vi "ECG AF SPI Input 2.vi"() -> ()   [LabVIEW 2017]
uses:
  ECG Data.ctl
  IBP Data.ctl
  Trigger Params.ctl
  Channel Enum.ctl
  <vilib>/Platform/TimedLoop/XDataNode/timing_clust.ctl
  <vilib>/Platform/TimedLoop/XDataNode/nitl_modes.ctl
  <vilib>/Platform/TimedLoop/XDataNode/wakeup.ctl
  Gradient Data.ctl
  All Data.ctl
  <vilib>/rvi/Emulation/niFpgaGetClockAttributes.vi
  <vilib>/rvi/Emulation/niFpgaSctlEmulationGetInTimedLoop.vi
  <vilib>/rvi/Emulation/niFpgaEmulationReportErrorSimple.vi
  <vilib>/rvi/DataTransferAndStorage/Container/Common/niFpgaContainerGetUniqueNameForEmu.vi
  <vilib>/rvi/DataTransferAndStorage/Container/Common/niFpgaContainerSetEmuInfo.vi
  <vilib>/rvi/eio/common/nirviEmuReportErrorAndStop.vi
  <vilib>/rvi/Emulation/niFpgaCriticalErrorInLSC.vi
  <vilib>/rvi/Emulation/niFpgaProcessEmulError.vi
  <vilib>/rvi/eio/common/nirviEmuTemplateMethod_errors.vi
  <vilib>/rvi/Analysis/common/codeGenErrors/XNode/niFpgaXNodeCodeGenErrorHandle.vi
  <vilib>/rvi/DataTransferAndStorage/Container/Common/niFpgaContainerExecOnDevCompGetState.vi
  <vilib>/rvi/Emulation/niFpgaEmulationIsFPGAContextNoSignature.vi
  <vilib>/rvi/errors/niFpgaSetErrorForExecOnDevCompSimple.vi
  <vilib>/rvi/FIFO/Fifo_Resource/nirvififoEmulationSetSize.vi
  <vilib>/rvi/FIFO/Fifo_Resource/nirviFifoEmulationQueueMgr.vi
  <instcachedir>/0/nirviFifoEmulationQueueMgr_E5CAEC123FF24DC58D834DCA3CDAA9B5.lvgen/nirviFifoEmulationQueueMgr_E5CAEC123FF24DC58D834DCA3CDAA9B5_002.vi
  <vilib>/rvi/FIFO/Fifo_Resource/nirvififoEmulationDetermineInputValidOut.vi
  <vilib>/rvi/FIFO/Fifo_Resource/nirvififoEmulationCreateLock.vi
  <vilib>/rvi/FIFO/Fifo_Resource/nirvififoEmulationObtainLock.vi
  <vilib>/rvi/FIFO/Fifo_Resource/nirvififoEmulationReleaseLock.vi
  <vilib>/rvi/occurrence/nirviWaitOnOccurrenceBase.vi
  <vilib>/rvi/errors/nirviReportUnexpectedCaseInternalError.vi
  <vilib>/rvi/errors/nirviReportUnexpectedCaseInternalError (U32).vi
  <vilib>/Utility/error.llb/Clear Errors.vi
  <vilib>/rvi/interface/RandomDataEmulation/niFpgaRandomDataHandleErrors.vi
  <instcachedir>/0/nirviFifoEmulationQueueMgr_E5CAEC123FF24DC58D834DCA3CDAA9B5.lvgen/nirviFifoEmulationQueueMgr_E5CAEC123FF24DC58D834DCA3CDAA9B5_003.vi
  <vilib>/Platform/TimedLoop/XDataNode/XDataNode.xnode
  <vilib>/rvi/LocalResourceManager/LocalResourceManager.xnode
  <vilib>/eio/EIONode/EIONode.xnode
  <vilib>/eio/EIOMethodNode/EIOMethodNode.xnode
  <vilib>/rvi/Analysis/measure/butterworth/XNode/niFpgaButterworthFilter.xnode
  <vilib>/rvi/Analysis/measure/LMRsmpl/XNode/niFPGA Rational Resampler.xnode
  <vilib>/rvi/DataTransferAndStorage/Container/XNode/niFpgaContainer.xnode
  <vilib>/rvi/FIFO/Fifo_Resource/niFpgaFifoEmulationRefIn.vi
  <vilib>/Platform/TimedLoop/XDataNode/XDNodeRunTimeDep.lvlib
panel:
  in  "Invert PWM IBP":bool
  in  "Invert PWM ECG":bool
  in  "IBP1":T1={"Scale"=1.0, "Offset"=0.0}
  in  "IBP0":T1={"Scale"=1.0, "Offset"=0.0}
  in  "IBP Filter":bool
  in  "Offset":cluster{"X":i16, "Y":i16, "Z":i16}
  in  "Beta IBP":fxp<+/-,32,-16>
  out "IPB0 In":i16
  out "IBP1 In":i16
  out "IPB0 Out":i16
  out "IBP1 Out":i16
  in  "ECG Scale":i16=1 min=1 max=100 step=1
  out "LL Out":i16
  out "LA Out":i16
  out "RA Out":i16
  out "LL In":i16
  out "LA In":i16
  out "RA In":i16
  in  "HPF":bool
  in  "Trigger":T2
  out "IBP Data":T4
  out "ECG Data":T5
  in  "Stop":bool
  in  "Reset":bool
  out "Send":bool
  out "WeightSum":fxp<+/-,33,19> format="%.20g"
  out "BetaProduct":fxp<+/-,32,-1> format="%.33g"
  out "Loop Time":u32
  in  "Filter Size":i16
  out "I In":i16
  out "II In":i16
  out "III In":i16
  out "aVR In":i16
  out "aVL In":i16
  out "aVF In":i16
  out "V1 In":i16
  out "V2 In":i16
  out "V3 In":i16
  out "V4 In":i16
  out "V5 In":i16
  out "V6 In":i16
  out "V4 Out":i16
  out "V5 Out":i16
  out "Trigger Out":i16
  out "IBP2":i16
  out "IBP1":i16
  out "IBP0":i16
  in  "Start":bool
  in  "Beta ECG":fxp<+/-,32,-16>
  out "V3 Out":i16
  out "V2 Out":i16
  out "V1 Out":i16
  out "aVF Out":i16
  out "aVL Out":i16
  out "aVR Out":i16
  out "III Out":i16
  out "II Out":i16
  out "I Out":i16
  out "V6":i16
  out "V5":i16
  out "V4":i16
  out "V3":i16
  out "V2":i16
  out "V1":i16
  out "LL":i16
  out "LA":i16
  out "Actual Loop Rate (Ticks)":u32
  out "Late? Latched":bool
  out "RA":i16
  in  "Loop Rate (Ticks)":u32=4000
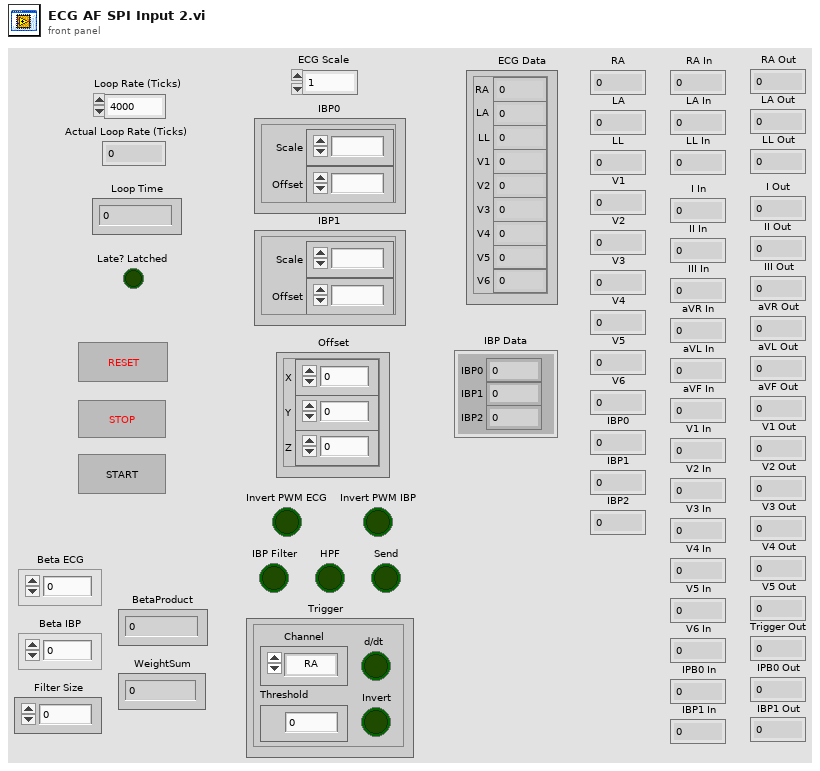
[diagram p1: front panel]
types:
  T1 = cluster{"Scale":fxp<+/-,16,5>, "Offset":fxp<+/-,16,16>}
  T2 = typedef "Trigger Params.ctl" = cluster{"Channel":T3, "Threshold":i16, "d/dt":bool, "Invert":bool}
  T3 = typedef "Channel Enum.ctl" = enum16{"RA", "LA", "LL", "V1", "V2", "V3", "V4", "V5", "V6", "I", "II", "III", "aVR", "aVL", "aVF", "Vw", "IBP1", "IBP2"}
  T4 = typedef "IBP Data.ctl" = cluster{"IBP0":fxp<+/-,16,16>, "IBP1":fxp<+/-,16,16>, "IBP2":fxp<+/-,16,16>}
  T5 = typedef "ECG Data.ctl" = cluster{"RA":fxp<+/-,16,16>, "LA":fxp<+/-,16,16>, "LL":fxp<+/-,16,16>, "V1":fxp<+/-,16,16>, "V2":fxp<+/-,16,16>, "V3":fxp<+/-,16,16>, "V4":fxp<+/-,16,16>, "V5":fxp<+/-,16,16>, "V6":fxp<+/-,16,16>}
  T6 = typedef "XDNodeRunTimeDep.lvlib/timing_clust.ctl" = cluster{"Expected End [f-1]":u64, "Actual End [f-1]":u64, "Finished Late? [f-1]":bool, "Expected End [i-1]":u64, "Actual End [i-1]":u64, "Finished Late? [i-1]":bool, "Expected Start [i]":u64, "Actual Start [i]":u64, "Expected Start [f]":u64, "Actual Start [f]":u64, "Source Name":string, "Structure Name":string, "Period":i64, "Deadline":i64, "Offset":i64, "Start":i64, "Priority":i32, "Timeout":i32, "Mode":T7, "Wakeup Reason":T8, "Error":errorcluster, "Source Type":string, "Secondary Source Type":string, "Global End Time":u64, "Global Start Time":u64, "Frame Duration":u64, "Iteration Duration":u64, "Assigned CPU":i32, "I/O Scan Engine Mode":u32}
  T7 = typedef "XDNodeRunTimeDep.lvlib/nitl_modes.ctl" = enum32{"No Change", "Process missed periods, maintain original phase", "Discard missed periods, maintain original phase", "Process missed periods, ignore original phase", "Discard missed periods, ignore original phase"}
  T8 = typedef "XDNodeRunTimeDep.lvlib/wakeup.ctl" = enum32{"Normal", "Aborted", "Asynchronous wakeup", "Timing source error", "Timed loop error", "Timeout"}
  T9 = typedef "Memory Block Channels.ctl" = cluster{"RA":T10, "LA":T10, "LL":T10, "V1":T10, "V2":T10, "V3":T10, "IBP0":T10, "IBP1":T10}
  T10 = typedef "MemoryBlocks.ctl" = cluster{"Taps":refnum<k21>, "Weights":refnum<k21>, "IO Weights":refnum<k21>, "IO Taps":refnum<k21>}
  T11 = cluster{"ECG":cluster{"RA":fxp<+/-,16,16>, "LA":fxp<+/-,16,16>, "LL":fxp<+/-,16,16>, "V1":fxp<+/-,16,16>, "V2":fxp<+/-,16,16>, "V3":fxp<+/-,16,16>, "V4":fxp<+/-,16,16>, "V5":fxp<+/-,16,16>, "V6":fxp<+/-,16,16>}, "Gradients":cluster{"X":fxp<+/-,16,16>, "Y":fxp<+/-,16,16>, "Z":fxp<+/-,16,16>}, "IBP":cluster{"IBP0":fxp<+/-,16,16>, "IBP1":fxp<+/-,16,16>, "IBP2":fxp<+/-,16,16>}}
  T12 = cluster{"BetaProduct":fxp<+/-,32,-1>, "WeightSum":fxp<+/-,33,19>}
  T13 = typedef "ECG Leads.ctl" = cluster{"RA":i16, "LA":i16, "LL":i16, "V1":i16, "V2":i16, "V3":i16, "V4":i16, "V5":i16, "Trigger":i16, "I":i16, "II":i16, "III":i16, "aVR":i16, "aVL":i16, "aVF":i16, "Vw":i16}
  T14 = cluster{"X":fxp<+/-,16,16>, "Y":fxp<+/-,16,16>, "Z":fxp<+/-,16,16>}
  T15 = cluster{"IBP0":fxp<+/-,16,16>, "IBP1":fxp<+/-,16,16>, "IBP2":fxp<+/-,16,16>}
  T16 = typedef "All Data.ctl" = cluster{"ECG":T5, "Gradients":T17, "IBP":T4}
  T17 = typedef "Gradient Data.ctl" = cluster{"X":fxp<+/-,16,16>, "Y":fxp<+/-,16,16>, "Z":fxp<+/-,16,16>}
  T18 = cluster{"[0]":fxp<+/-,16,16>, "[1]":fxp<+/-,16,16>, "[2]":fxp<+/-,16,16>}
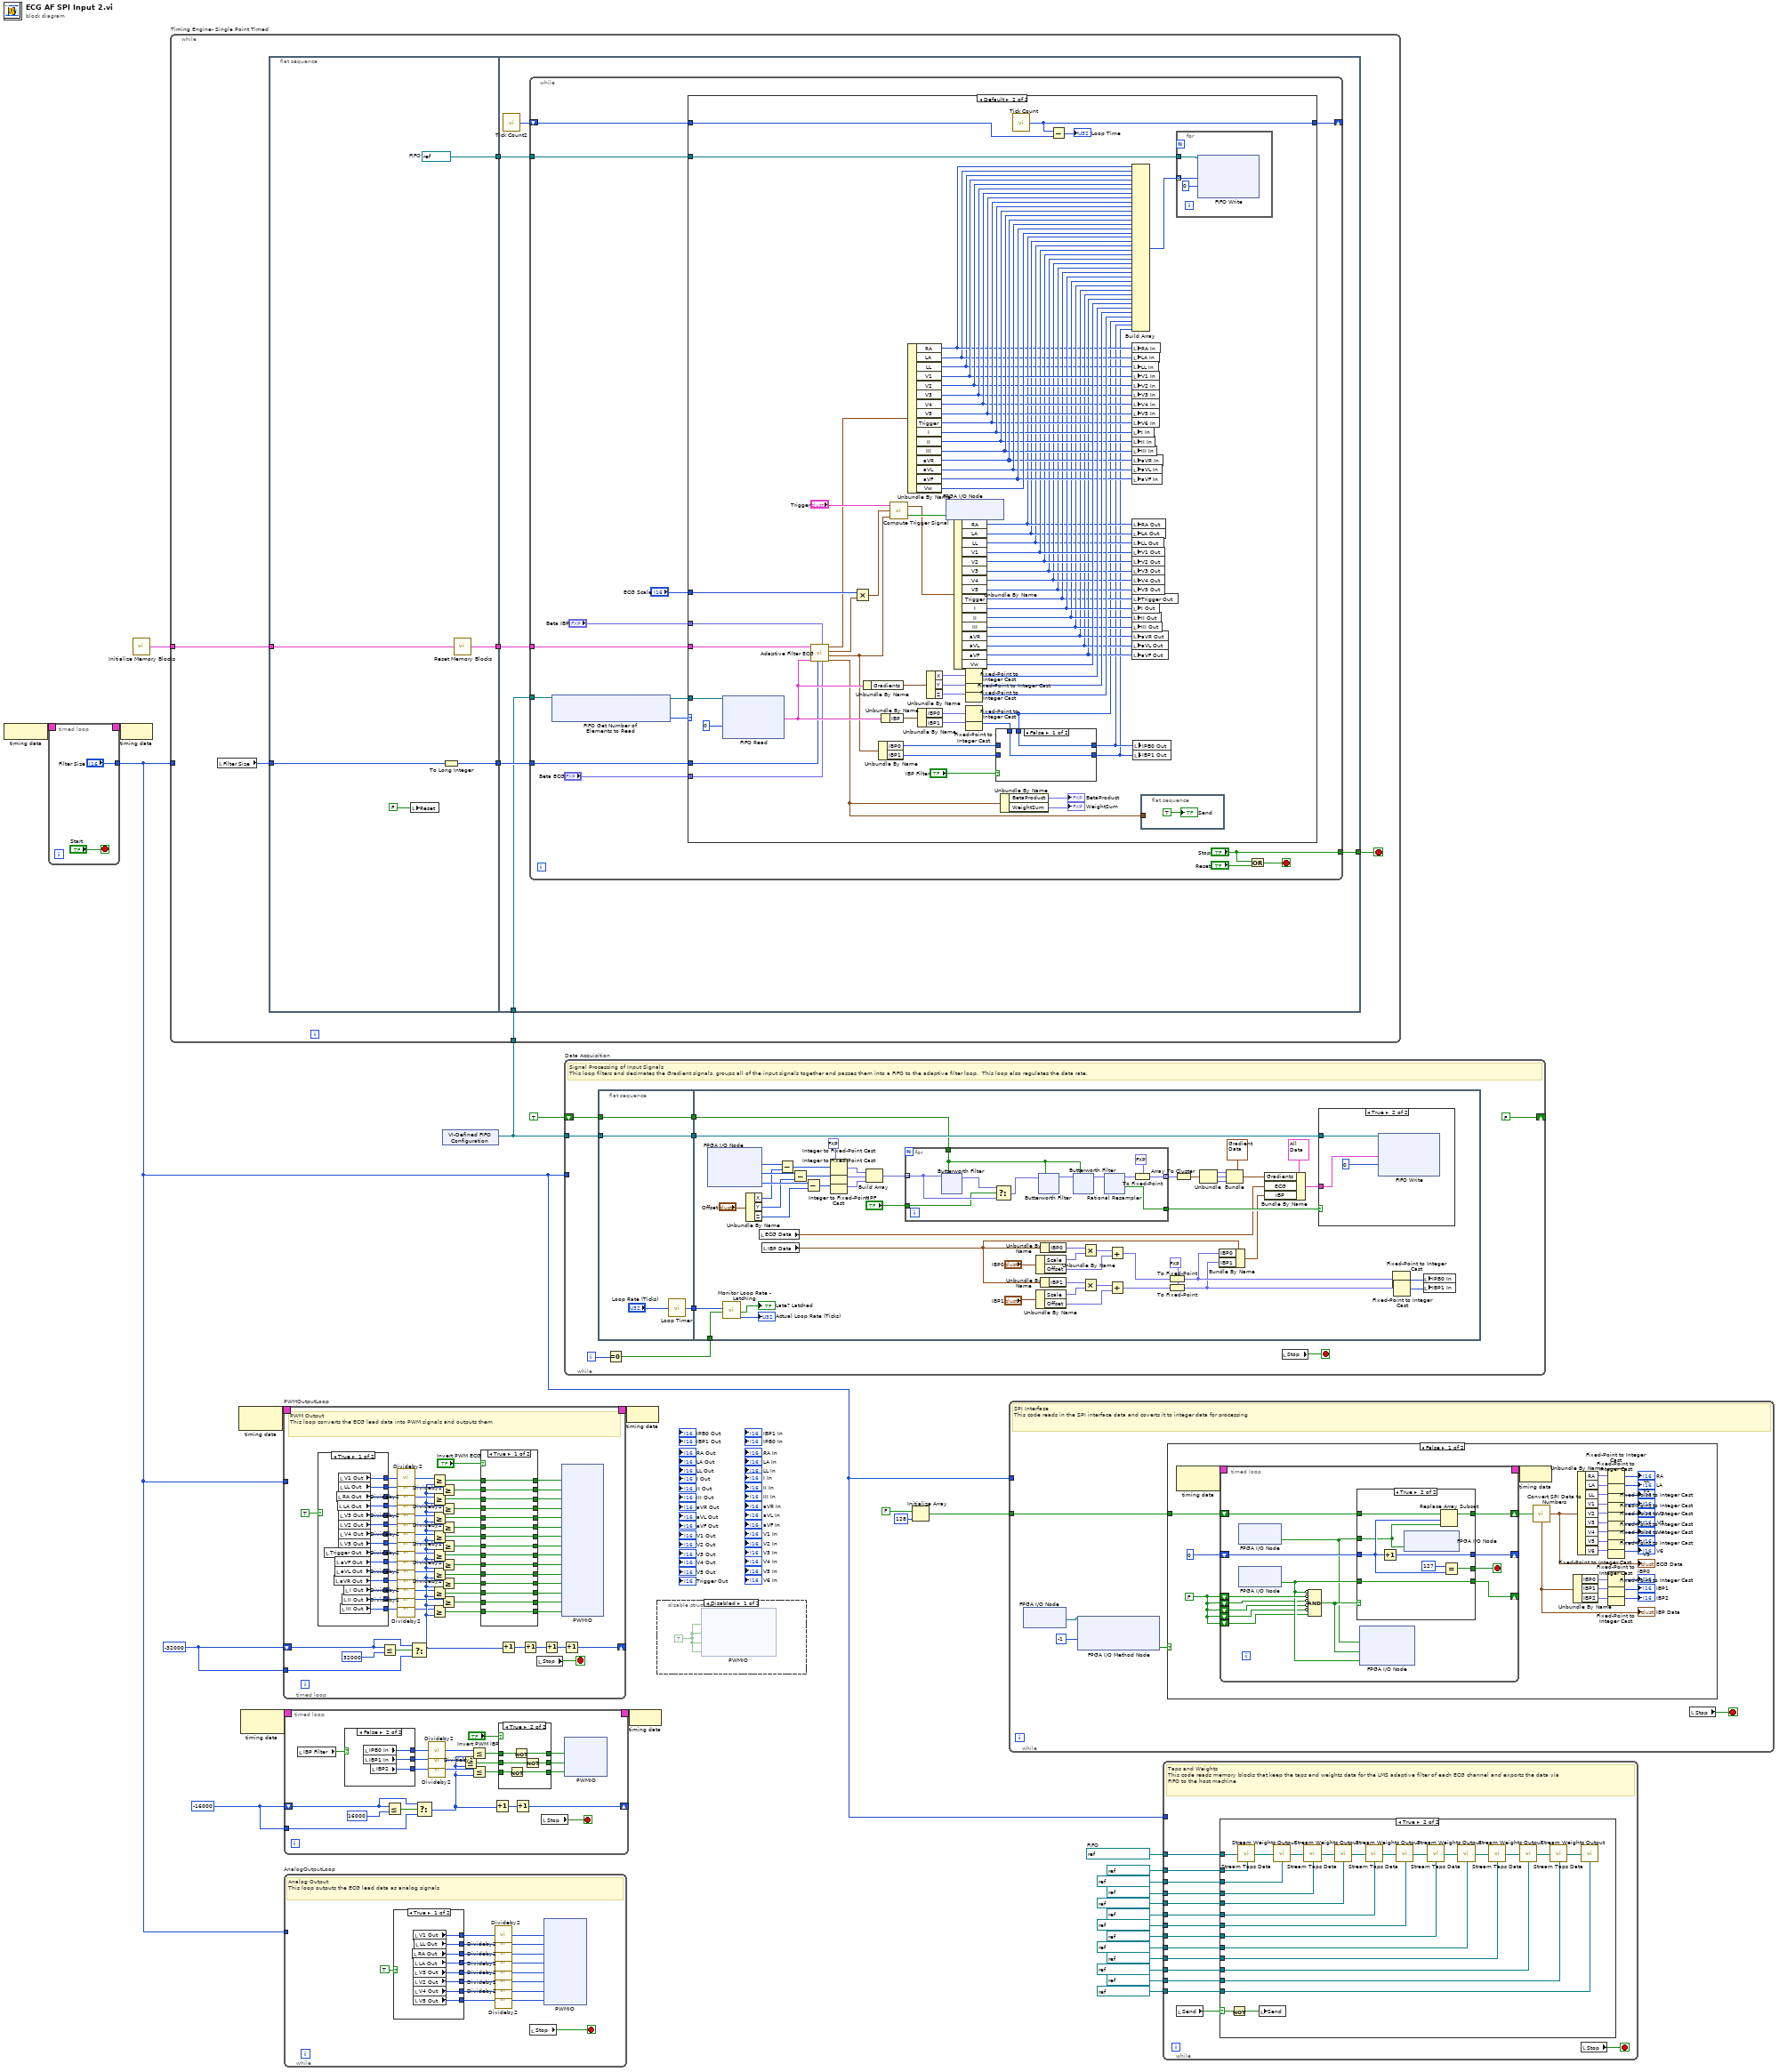
[diagram p0: block diagram]
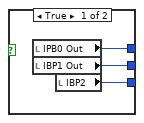
[diagram p4: hidden frame]
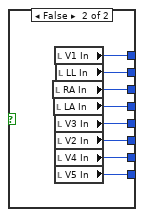
[diagram p7: hidden frame]
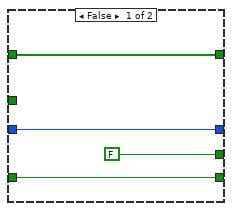
[diagram p8: hidden frame]
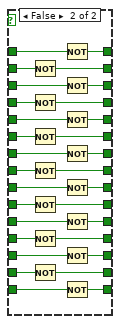
[diagram p10: hidden frame]
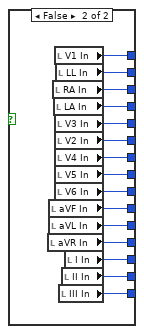
[diagram p11: hidden frame]
diagram:
  w1 = i16 -16000
  w10 = refnum<k21> "FIFO Filter Specs"  # FIFO
  w26 = i16 -32000
  n1 = node-c288 ("Input Node")() -> (w7:T6)
  n2 = timed-loop "initWait" {
    timing: w7 -> [_]
    timing-out: [_] -> w6
    tunnel: ["Filter Size"] -> w5
    stop <- "Start" stop-if-true
  }
  n3 = node-c288 ("Output Node")(w6) -> ()
  n4 = call "Initialize Memory Blocks.vi"() -> ("Memory"=w9:T9)
  n5 = node-c288 ("Input Node")() -> (w28:T6)  [unwired: 1 in]
  n6 = node-c288() -> (w3:T6)  [unwired: 1 in]
  n7 = timed-loop "PWMOutputLoop" {
    timing: w28 -> [_]
    timing-out: [_] -> w27
    shift-right: [w95] -> _
    shift-left: w26 -> [w102]
    tunnel: w26 -> [w100]
    tunnel: w5 -> [_]
    stop <- w72 stop-if-true
    # "PWM Output\nThis loop converts the ECG lead data into PWM signals and outputs them"
    n8 = case shown="True" TRUE {
      tunnel: [w164 w179] -> w98
      tunnel: [w163 w178] -> w97
      tunnel: [w162 w177] -> w91
      tunnel: [w161 w176] -> w92
      tunnel: [w160 w175] -> w88
      tunnel: [w159 w174] -> w87
      tunnel: [w158 w173] -> w89
      tunnel: [w157 w172] -> w90
      tunnel: [w156 w171] -> w86
      tunnel: [w155 w170] -> w78
      tunnel: [w154 w169] -> w77
      tunnel: [w153 w168] -> w76
      tunnel: [w152 w167] -> w71
      tunnel: [w151 w166] -> w70
      tunnel: [w150 w165] -> w69
      frame True {
        n9 = local read "Trigger Out"() -> (w156:i16)
        n10 = local read "aVR Out"() -> (w153:i16)
        n11 = local read "aVF Out"() -> (w155:i16)
        n12 = local read "aVL Out"() -> (w154:i16)
        n13 = local read "RA Out"() -> (w161:i16)
        n14 = local read "LA Out"() -> (w162:i16)
        n15 = local read "V1 Out"() -> (w164:i16)
        n16 = local read "V3 Out"() -> (w157:i16)
        n17 = local read "V2 Out"() -> (w158:i16)
        n18 = local read "V4 Out"() -> (w160:i16)
        n19 = local read "V5 Out"() -> (w159:i16)
        n20 = local read "LL Out"() -> (w163:i16)
        n21 = local read "III Out"() -> (w150:i16)
        n22 = local read "II Out"() -> (w151:i16)
        n23 = local read "I Out"() -> (w152:i16)
      }
      frame False {
        n24 = local read "aVR In"() -> (w168:i16)
        n25 = local read "aVF In"() -> (w170:i16)
        n26 = local read "aVL In"() -> (w169:i16)
        n27 = local read "RA In"() -> (w176:i16)
        n28 = local read "LA In"() -> (w177:i16)
        n29 = local read "V1 In"() -> (w179:i16)
        n30 = local read "V3 In"() -> (w172:i16)
        n31 = local read "V2 In"() -> (w173:i16)
        n32 = local read "V4 In"() -> (w175:i16)
        n33 = local read "V5 In"() -> (w174:i16)
        n34 = local read "V6 In"() -> (w171:i16)
        n35 = local read "LL In"() -> (w178:i16)
        n36 = local read "III In"() -> (w165:i16)
        n37 = local read "II In"() -> (w166:i16)
        n38 = local read "I In"() -> (w167:i16)
      }
    }
    n39 = Less Or Equal?(x=w102, y=i16 32000 ("Period")) -> (x <= y?=w103:bool)
    n40 = call "Divideby2.vi"("Input"=w98) -> ("Output"=w94:i16)
    n41 = call "Divideby2.vi"("Input"=w97) -> ("Output"=w93:i16)
    n42 = call "Divideby2.vi"("Input"=w92) -> ("Output"=w79:i16)
    n43 = call "Divideby2.vi"("Input"=w91) -> ("Output"=w80:i16)
    n44 = call "Divideby2.vi"("Input"=w90) -> ("Output"=w81:i16)
    n45 = call "Divideby2.vi"("Input"=w89) -> ("Output"=w82:i16)
    n46 = call "Divideby2.vi"("Input"=w88) -> ("Output"=w83:i16)
    n47 = call "Divideby2.vi"("Input"=w87) -> ("Output"=w84:i16)
    n48 = call "Divideby2.vi"("Input"=w86) -> ("Output"=w85:i16)
    n49 = call "Divideby2.vi"("Input"=w78) -> ("Output"=w75:i16)
    n50 = call "Divideby2.vi"("Input"=w77) -> ("Output"=w74:i16)
    n51 = call "Divideby2.vi"("Input"=w76) -> ("Output"=w73:i16)
    n52 = call "Divideby2.vi"("Input"=w71) -> ("Output"=w66:i16)
    n53 = call "Divideby2.vi"("Input"=w70) -> ("Output"=w67:i16)
    n54 = call "Divideby2.vi"("Input"=w69) -> ("Output"=w65:i16)
    n55 = Select(t=w102, s=w103, f=w100) -> (s? t:f=w68:i16)
    n56 = Greater Or Equal?(x=w94, y=w68) -> (x >= y?=w62:bool)
    n57 = Greater Or Equal?(x=w79, y=w68) -> (x >= y?=w60:bool)
    n58 = Greater Or Equal?(x=w81, y=w68) -> (x >= y?=w58:bool)
    n59 = Greater Or Equal?(x=w83, y=w68) -> (x >= y?=w56:bool)
    n60 = Greater Or Equal?(x=w85, y=w68) -> (x >= y?=w54:bool)
    n61 = Greater Or Equal?(x=w74, y=w68) -> (x >= y?=w52:bool)
    n62 = Greater Or Equal?(x=w66, y=w68) -> (x >= y?=w50:bool)
    n63 = Greater Or Equal?(x=w65, y=w68) -> (x >= y?=w48:bool)
    n64 = Greater Or Equal?(x=w93, y=w68) -> (x >= y?=w61:bool)
    n65 = Greater Or Equal?(x=w80, y=w68) -> (x >= y?=w59:bool)
    n66 = Greater Or Equal?(x=w82, y=w68) -> (x >= y?=w57:bool)
    n67 = Greater Or Equal?(x=w84, y=w68) -> (x >= y?=w55:bool)
    n68 = Greater Or Equal?(x=w75, y=w68) -> (x >= y?=w53:bool)
    n69 = Greater Or Equal?(x=w73, y=w68) -> (x >= y?=w51:bool)
    n70 = Greater Or Equal?(x=w67, y=w68) -> (x >= y?=w49:bool)
    n71 = case shown="True" "Invert PWM ECG" {
      tunnel: w62 -> [w119 w149]
      tunnel: w61 -> [w118 w148]
      tunnel: w60 -> [w117 w147]
      tunnel: w59 -> [w116 w146]
      tunnel: w58 -> [w115 w145]
      tunnel: w57 -> [w114 w144]
      tunnel: w56 -> [w113 w143]
      tunnel: w55 -> [w112 w142]
      tunnel: w54 -> [w111 w141]
      tunnel: w53 -> [w110 w140]
      tunnel: w52 -> [w109 w139]
      tunnel: w51 -> [w108 w138]
      tunnel: w50 -> [w107 w137]
      tunnel: w49 -> [w106 w136]
      tunnel: w48 -> [w105 w135]
      tunnel: [w119 w134] -> w47
      tunnel: [w118 w133] -> w46
      tunnel: [w117 w132] -> w45
      tunnel: [w116 w131] -> w44
      tunnel: [w115 w130] -> w43
      tunnel: [w114 w129] -> w42
      tunnel: [w113 w128] -> w41
      tunnel: [w112 w127] -> w40
      tunnel: [w111 w126] -> w39
      tunnel: [w110 w125] -> w38
      tunnel: [w109 w124] -> w37
      tunnel: [w108 w123] -> w36
      tunnel: [w107 w122] -> w35
      tunnel: [w106 w121] -> w34
      tunnel: [w105 w120] -> w33
      frame True {
      }
      frame False {
        n72 = Not(x=w148) -> (.not. x?=w133:bool)
        n73 = Not(x=w146) -> (.not. x?=w131:bool)
        n74 = Not(x=w144) -> (.not. x?=w129:bool)
        n75 = Not(x=w142) -> (.not. x?=w127:bool)
        n76 = Not(x=w140) -> (.not. x?=w125:bool)
        n77 = Not(x=w138) -> (.not. x?=w123:bool)
        n78 = Not(x=w136) -> (.not. x?=w121:bool)
        n79 = Not(x=w149) -> (.not. x?=w134:bool)
        n80 = Not(x=w147) -> (.not. x?=w132:bool)
        n81 = Not(x=w145) -> (.not. x?=w130:bool)
        n82 = Not(x=w143) -> (.not. x?=w128:bool)
        n83 = Not(x=w141) -> (.not. x?=w126:bool)
        n84 = Not(x=w139) -> (.not. x?=w124:bool)
        n85 = Not(x=w137) -> (.not. x?=w122:bool)
        n86 = Not(x=w135) -> (.not. x?=w120:bool)
      }
    }
    n87 = Increment(x=w68) -> (x+1=w101:i16)
    n88 = Increment(x=w101) -> (x+1=w99:i16)
    n89 = local read "Stop"() -> (w72:bool)
    n90 = Increment(x=w99) -> (x+1=w96:i16)
    n91 = xnode ("PWMIO")("V1"=w47, "LL"=w46, "RA"=w45, "LA"=w44, "V3"=w43, "V2"=w42, "V4"=w41, "V5"=w40, "V6"=w39, "aVF"=w38, "aVL"=w37, "aVR"=w36, "I"=w35, "II"=w34, "III"=w33) -> ()  [unwired: 15 in, 15 out]
    n92 = Increment(x=w96) -> (x+1=w95:i16)
  }
  n93 = while "AnalogOutputLoop" {
    tunnel: w5 -> [_]
    stop <- w196 stop-if-true
    # "Analog Output\nThis loop outputs the ECG lead data as analog signals"
    n94 = case shown="True" TRUE {
      tunnel: [w207 w215] -> w198
      tunnel: [w206 w214] -> w197
      tunnel: [w205 w213] -> w199
      tunnel: [w200 w212] -> w187
      tunnel: [w201 w211] -> w186
      tunnel: [w202 w210] -> w185
      tunnel: [w203 w209] -> w184
      tunnel: [w204 w208] -> w183
      frame True {
        n95 = local read "RA Out"() -> (w202:i16)
        n96 = local read "LA Out"() -> (w201:i16)
        n97 = local read "V1 Out"() -> (w204:i16)
        n98 = local read "V3 Out"() -> (w200:i16)
        n99 = local read "V2 Out"() -> (w205:i16)
        n100 = local read "V4 Out"() -> (w207:i16)
        n101 = local read "V5 Out"() -> (w206:i16)
        n102 = local read "LL Out"() -> (w203:i16)
      }
      frame False {
        n103 = local read "RA In"() -> (w210:i16)
        n104 = local read "LA In"() -> (w211:i16)
        n105 = local read "V1 In"() -> (w208:i16)
        n106 = local read "V3 In"() -> (w212:i16)
        n107 = local read "V2 In"() -> (w213:i16)
        n108 = local read "V4 In"() -> (w215:i16)
        n109 = local read "V5 In"() -> (w214:i16)
        n110 = local read "LL In"() -> (w209:i16)
      }
    }
    n111 = call "Divideby2.vi"("Input"=w183) -> ("Output"=w195:i16)
    n112 = call "Divideby2.vi"("Input"=w184) -> ("Output"=w194:i16)
    n113 = call "Divideby2.vi"("Input"=w185) -> ("Output"=w193:i16)
    n114 = call "Divideby2.vi"("Input"=w186) -> ("Output"=w192:i16)
    n115 = call "Divideby2.vi"("Input"=w187) -> ("Output"=w191:i16)
    n116 = call "Divideby2.vi"("Input"=w199) -> ("Output"=w190:i16)
    n117 = call "Divideby2.vi"("Input"=w198) -> ("Output"=w189:i16)
    n118 = call "Divideby2.vi"("Input"=w197) -> ("Output"=w188:i16)
    n119 = local read "Stop"() -> (w196:bool)
    n120 = xnode ("PWMIO")("ECG0"=w195, "ECG1"=w194, "ECG2"=w193, "ECG3"=w192, "ECG4"=w191, "ECG5"=w190, "ECG6"=w189, "ECG7"=w188) -> ()  [unwired: 8 in, 8 out]
  }
  n121 = timed-loop {
    timing: w3 -> [_]
    timing-out: [_] -> w2
    shift-right: [w223] -> _
    shift-left: w1 -> [w229]
    tunnel: w1 -> [w227]
    stop <- w228 stop-if-true
    n122 = local read "IBP Filter"() -> (w226:bool)
    n123 = case shown="False" w226 {
      tunnel: [w249 w252] -> w234
      tunnel: [w248 w251] -> w233
      tunnel: [w247 w250] -> w232
      frame True {
        n124 = local read "IPB0 Out"() -> (w249:i16)
        n125 = local read "IBP1 Out"() -> (w248:i16)
        n126 = local read "IBP2"() -> (w247:i16)
      }
      frame False {
        n127 = local read "IPB0 In"() -> (w252:i16)
        n128 = local read "IBP1 In"() -> (w251:i16)
        n129 = local read "IBP2"() -> (w250:i16)
      }
    }
    n130 = Less Or Equal?(x=w229, y=i16 16000 ("Period")) -> (x <= y?=w231:bool)
    n131 = Select(t=w229, s=w231, f=w227) -> (s? t:f=w225:i16)
    n132 = call "Divideby2.vi"("Input"=w234) -> ("Output"=w237:i16)
    n133 = call "Divideby2.vi"("Input"=w233) -> ("Output"=w236:i16)
    n134 = call "Divideby2.vi"("Input"=w232) -> ("Output"=w235:i16)
    n135 = Less Or Equal?(x=w236, y=w225) -> (x <= y?=w220:bool)
    n136 = Less Or Equal?(x=w237, y=w225) -> (x <= y?=w221:bool)
    n137 = Less Or Equal?(x=w235, y=w225) -> (x <= y?=w219:bool)
    n138 = Increment(x=w225) -> (x+1=w224:i16)
    n139 = case shown="True" "Invert PWM IBP" {
      tunnel: w221 -> [w240 w246]
      tunnel: w220 -> [w239 w245]
      tunnel: w219 -> [w238 w244]
      tunnel: [w240 w243] -> w218
      tunnel: [w239 w242] -> w217
      tunnel: [w238 w241] -> w216
      frame False {
      }
      frame True {
        n140 = Not(x=w244) -> (.not. x?=w241:bool)
        n141 = Not(x=w246) -> (.not. x?=w243:bool)
        n142 = Not(x=w245) -> (.not. x?=w242:bool)
      }
    }
    n143 = Increment(x=w224) -> (x+1=w223:i16)
    n144 = local read "Stop"() -> (w228:bool)
    n145 = xnode ("PWMIO")("IBP0"=w218, "IBP1"=w217, "IBP2"=w216) -> ()  [unwired: 3 in, 3 out]
  }
  n146 = xnode "VI-Defined FIFO Configuration"() -> ("FIFO Out"=w8:refnum<k21>)
  n147 = while "Timing Engine- Single Point Timed" {
    tunnel: w9 -> [w257]
    tunnel: w8 -> [w256]
    tunnel: w5 -> [_]
    stop <- w258 stop-if-true
    n148 = local read "Filter Size"() -> (w255:i16)
    n149 = flat-sequence "MainSeq" {
      tunnel: [w267] -> w261
      tunnel: [w266] -> w260
      tunnel: [w265] -> w259
      tunnel: w257 -> [w264]
      tunnel: w255 -> [w263]
      tunnel: w261 -> [w273]
      tunnel: w260 -> [w272]
      tunnel: w259 -> [w271]
      tunnel: [w269] -> w258
      tunnel: w256 -> [w268]
      frame #0 {
        w267 = refnum<k21> "FIFO"  # FIFO
        n150 = local write "Reset"(FALSE ("Reset")) -> ()
        n151 = To Long Integer(number=w263) -> (32bit integer=w266:i32)
        n152 = call "Reset Memory Blocks.vi"("Memory Blocks In"=w264) -> ("Memory Blocks Out"=w265:T9)  [unwired: 1 in]
      }
      frame #1 {
        n153 = call "Tick Count2"() -> ("Tick Count(uSec)"=w270:u32)
        n154 = while {
          tunnel: w268 -> [w287]
          tunnel: w273 -> [w283]
          tunnel: w272 -> [w282]
          tunnel: w271 -> [w276]
          shift-right: [w281] -> _
          shift-left: w270 -> [w280]
          tunnel: ["Stop"] -> w269
          stop <- w278 stop-if-true
          n155 = xnode ("FIFO Get Number of Elements to Read")("FIFO In"=w287) -> ("Number of Elements to Read"=w286:u32, "FIFO Out"=w285:refnum<k21>)
          n156 = case shown="Default" w286 {
            tunnel: w285 -> [_ w360]
            tunnel: "Beta ECG" -> [_ w312]
            tunnel: w283 -> [_ w358]
            tunnel: w282 -> [_ w313]
            tunnel: w280 -> [w288 w322]
            tunnel: [w288 w323] -> w281
            tunnel: w276 -> [_ w319]
            tunnel: "ECG Scale" -> [_ w302]
            tunnel: "Beta IBP" -> [_ w299]
            frame 0 {
            }
            frame Default {
              n157 = xnode ("FIFO Read")("Timeout"=0, "FIFO In"=w360) -> ("Element"=w315:T11)  [unwired: 2 out]
              n158 = call "Adaptive Filter ECG.vi"("Beta"=w312, "Beta IBP"=w299, "Filter Length"=w313, "Data in"=w315, "Memory Blocks In"=w319) -> ("Data"=w314:T12, "IBP Out"=w298:cluster{"IBP0":i16, "IBP1":i16}, "Filtered Leads"=w303:T13, "Raw Leads"=w300:T13)  [unwired: 3 in]
              n159 = Multiply(x=w302, y=w303) -> (x*y=w301:T13)
              n160 = Unbundle By Name(w315) -> ("Gradients"=w318:T14)
              n161 = Unbundle By Name(w298) -> ("IBP0"=w294:i16, "IBP1"=w295:i16)
              n162 = Unbundle By Name(w315) -> ("IBP"=w317:T15)
              n163 = call "Compute Trigger Signal.vi"("IBP Out"=w298, "Filtered Leads"=w301, "Trigger"="Trigger") -> ("Trigger Out"=w310:bool, "Leads Out"=w289:T13)
              n164 = Unbundle By Name(w300) -> ("RA"=w306:i16, "LA"=w305:i16, "LL"=w304:i16, "V1"=w337:i16, "V2"=w338:i16, "V3"=w339:i16, "V4"=w340:i16, "V5"=w341:i16, "Trigger"=w342:i16, "I"=w343:i16, "II"=w344:i16, "III"=w345:i16, "aVR"=w346:i16, "aVL"=w347:i16, "aVF"=w348:i16, "Vw"=w353:i16)
              n165 = Unbundle By Name(w317) -> ("IBP0"=w316:fxp<+/-,16,16>, "IBP1"=w297:fxp<+/-,16,16>)
              n166 = Unbundle By Name(w318) -> ("X"=w356:fxp<+/-,16,16>, "Y"=w355:fxp<+/-,16,16>, "Z"=w354:fxp<+/-,16,16>)
              n167 = xnode "FPGA I/O Node"("Trigger Out"=w310) -> ()  [unwired: 1 in, 1 out]
              n168 = Unbundle By Name(w289) -> ("RA"=w309:i16, "LA"=w308:i16, "LL"=w307:i16, "V1"=w336:i16, "V2"=w335:i16, "V3"=w334:i16, "V4"=w333:i16, "V5"=w325:i16, "Trigger"=w326:i16, "I"=w332:i16, "II"=w331:i16, "III"=w330:i16, "aVR"=w329:i16, "aVL"=w328:i16, "aVF"=w327:i16, "Vw"=w352:i16)
              n169 = Fixed-Point to Integer Cast(1:w356) -> (0:w351:i16)
              n170 = Fixed-Point to Integer Cast(1:w355) -> (0:w350:i16)
              n171 = Fixed-Point to Integer Cast(1:w354) -> (0:w349:i16)
              n172 = Fixed-Point to Integer Cast(1:w316) -> (0:w290:i16)
              n173 = Fixed-Point to Integer Cast(1:w297) -> (0:w291:i16)
              n174 = case shown="False" "IBP Filter" {
                tunnel: w295 -> [_ w363]
                tunnel: w294 -> [_ w364]
                tunnel: [w361 w364] -> w293
                tunnel: [w362 w363] -> w292
                tunnel: w291 -> [w362 _]
                tunnel: w290 -> [w361 _]
                frame False {
                }
                frame True {
                }
              }
              n175 = Unbundle By Name(w314) -> ("BetaProduct"=→"BetaProduct":fxp<+/-,32,-1>, "WeightSum"=→"WeightSum":fxp<+/-,33,19>)
              n176 = call "Tick Count"() -> ("Tick Count(uSec)"=w323:u32)
              n177 = Subtract(x=w323, y=w322) -> (x-y=→"Loop Time":u32)
              n178 = Build Array(w306, w305, w304, w337, w338, w339, w340, w341, w342, w343, w344, w345, w346, w347, w348, w353, w309, w308, w307, w336, w335, w334, w333, w325, w326, w332, w331, w330, w329, w328, w327, w352, w351, w350, w349, w290, w293, w292) -> (w357:i16[])
              n179 = local write "RA In"(w306) -> ()
              n180 = local write "LA In"(w305) -> ()
              n181 = local write "LL In"(w304) -> ()
              n182 = local write "V1 In"(w337) -> ()
              n183 = local write "V2 In"(w338) -> ()
              n184 = local write "V3 In"(w339) -> ()
              n185 = local write "V4 In"(w340) -> ()
              n186 = local write "V5 In"(w341) -> ()
              n187 = local write "V6 In"(w342) -> ()
              n188 = local write "I In"(w343) -> ()
              n189 = local write "II In"(w344) -> ()
              n190 = local write "III In"(w345) -> ()
              n191 = local write "aVR In"(w346) -> ()
              n192 = local write "aVL In"(w347) -> ()
              n193 = local write "aVF In"(w348) -> ()
              n194 = local write "RA Out"(w309) -> ()
              n195 = local write "LA Out"(w308) -> ()
              n196 = local write "LL Out"(w307) -> ()
              n197 = local write "V1 Out"(w336) -> ()
              n198 = local write "V2 Out"(w335) -> ()
              n199 = local write "V3 Out"(w334) -> ()
              n200 = local write "V4 Out"(w333) -> ()
              n201 = local write "V5 Out"(w325) -> ()
              n202 = local write "Trigger Out"(w326) -> ()
              n203 = local write "I Out"(w332) -> ()
              n204 = local write "II Out"(w331) -> ()
              n205 = local write "III Out"(w330) -> ()
              n206 = local write "aVR Out"(w329) -> ()
              n207 = local write "aVL Out"(w328) -> ()
              n208 = local write "aVF Out"(w327) -> ()
              n209 = local write "IPB0 Out"(w293) -> ()
              n210 = local write "IBP1 Out"(w292) -> ()
              n211 = flat-sequence {
                tunnel: w314 -> [_]
                frame #0 {
                  "Send" <- TRUE ("Send")
                }
              }
              n212 = for {
                tunnel: w358 -> [w368]
                tunnel: w357 -> [w366] mode=indexing
                n213 = xnode ("FIFO Write")("Element"=w366, "Timeout"=0, "FIFO In"=w368) -> ()  [unwired: 2 out]
              }
            }
          }
          n214 = Or(x="Stop", y="Reset") -> (x .or. y?=w278:bool)
        }
      }
    }
  }
  n215 = while "Data Acquisition" {
    tunnel: w8 -> [w376]
    tunnel: w5 -> [_]
    shift-right: [FALSE] -> _
    shift-left: TRUE -> [w371]
    i -> [w374]
    stop <- w372 stop-if-true
    # "Signal Processing of Input Signals\nThis loop filters and decimates the Gradient signals, groups all of the input signals together and passes them into a FIFO to the adaptive filter loop.  This loop also regulates the data rate."
    n216 = flat-sequence "Data Acquisition Sequence" {
      tunnel: ["Loop Rate (Ticks)"] -> w377
      tunnel: w376 -> [w380]
      tunnel: [w380] -> w375
      tunnel: w371 -> [w378]
      tunnel: [w378] -> w370
      tunnel: w377 -> [w430]
      tunnel: w373 -> [w431]
      tunnel: w375 -> [w429]
      tunnel: w370 -> [w408]
      frame #0 {
        n217 = call "Loop Timer"("Count(Ticks)"="Loop Rate (Ticks)") -> ()  [unwired: 1 out]
      }
      frame #1 {
        w393 = fxp<+/-,16,16> 0.0 ("IBP Scale")
        w419 = fxp<+/-,16,16> 0.0 ("fixed-point type")
        n218 = xnode "FPGA I/O Node"() -> ("X Gradient"=w422:i16, "Y Gradient"=w421:i16, "Z Gradient"=w420:i16)  [unwired: 3 in, 3 out]
        n219 = call "Monitor Loop Rate - Latching.vi"("Reset"=w431, "Count(Ticks)"=w430) -> ("Actual Loop Rate (Ticks)"=→"Actual Loop Rate (Ticks)":u32, "Late? (Latched)"=→"Late? Latched":bool)  [unwired: 7 in, 1 out]
        n220 = Unbundle By Name("Offset") -> ("X"=w402:i16, "Y"=w400:i16, "Z"=w398:i16)
        n221 = local read "ECG Data"() -> (w409:T5)
        n222 = local read "IBP Data"() -> (w383:T4)
        n223 = Subtract(x=w422, y=w402) -> (x-y=w403:i16)
        n224 = Subtract(x=w421, y=w400) -> (x-y=w401:i16)
        n225 = Subtract(x=w420, y=w398) -> (x-y=w399:i16)
        n226 = Integer to Fixed-Point Cast(fixed-point type=w419, integer=w403) -> (fixed-point=w424:fxp<+/-,16,16>)
        n227 = Integer to Fixed-Point Cast(fixed-point type=w419, integer=w401) -> (fixed-point=w425:fxp<+/-,16,16>)
        n228 = Integer to Fixed-Point Cast(fixed-point type=w419, integer=w399) -> (fixed-point=w423:fxp<+/-,16,16>)
        n229 = Build Array(w424, w425, w423) -> (w426:fxp<+/-,16,16>[])
        n230 = for {
          tunnel: w426 -> [w435] mode=indexing
          tunnel: [w439] -> w418 mode=indexing
          tunnel: [w440] -> w428
          tunnel: w408 -> [w437]
          tunnel: "HPF" -> [w433]
          n231 = xnode "Butterworth Filter"("input data"=w435, "reset"=w437) -> ("output data"=w436:fxp<+/-,16,16>)  [unwired: 1 in, 1 out]
          n232 = Select(t=w436, s=w433, f=w435) -> (s? t:f=w434:fxp<+/-,16,16>)
          n233 = xnode "Butterworth Filter"("input data"=w434, "reset"=w437) -> ("output data"=w443:fxp<+/-,16,16>)  [unwired: 1 in, 1 out]
          n234 = xnode "Butterworth Filter"("input data"=w443, "reset"=w437) -> ("output data"=w442:fxp<+/-,16,16>)  [unwired: 1 in, 1 out]
          n235 = xnode "Rational Resampler"("input data"=w442) -> ("output data"=w441:fxp<+/-,18,16>, "output valid"=w440:bool)  [unwired: 1 out]
          n236 = To Fixed-Point(fixed-point type=fxp<+/-,16,16> 0.0, number=w441) -> (fixed-point=w439:fxp<+/-,16,16>)
        }
        n237 = Unbundle By Name("IBP0") -> ("Scale"=w391:fxp<+/-,16,5>, "Offset"=w389:fxp<+/-,16,16>)
        n238 = Unbundle By Name("IBP1") -> ("Scale"=w385:fxp<+/-,16,5>, "Offset"=w387:fxp<+/-,16,16>)
        n239 = Unbundle By Name(w383) -> ("IBP0"=w390:fxp<+/-,16,16>)
        n240 = Unbundle By Name(w383) -> ("IBP1"=w386:fxp<+/-,16,16>)
        n241 = Multiply(x=w390, y=w391) -> (x*y=w397:fxp<+/-,32,21>)
        n242 = Multiply(x=w386, y=w385) -> (x*y=w384:fxp<+/-,32,21>)
        n243 = Add(x=w397, y=w389) -> (x+y=w388:fxp<+/-,32,21>)
        n244 = Add(x=w384, y=w387) -> (x+y=w381:fxp<+/-,32,21>)
        n245 = To Fixed-Point(fixed-point type=w393, number=w388) -> (fixed-point=w396:fxp<+/-,16,16>)
        n246 = To Fixed-Point(fixed-point type=w393, number=w381) -> (fixed-point=w394:fxp<+/-,16,16>)
        n247 = Array To Cluster(array=w418) -> (cluster=w417:T18)
        n248 = Unbundle(w417) -> ("[0]"=w415:fxp<+/-,16,16>, "[1]"=w414:fxp<+/-,16,16>, "[2]"=w413:fxp<+/-,16,16>)
        n249 = Bundle By Name(cluster=w383, "IBP0"=w396, "IBP1"=w394) -> (w395:T4)
        n250 = Bundle(cluster=T17 {"X"=0.0, "Y"=0.0, "Z"=0.0} ("Gradients"), "X"=w415, "Y"=w414, "Z"=w413) -> (w411:T17)
        n251 = Bundle By Name(cluster=T16 {"ECG"={"RA"=0.0, "LA"=0.0, "LL"=0.0, "V1"=0.0, "V2"=0.0, "V3"=0.0, "V4"=0.0, "V5"=0.0, "V6"=0.0}, "Gradients"={"X"=0.0, "Y"=0.0, "Z"=0.0}, "IBP"={"IBP0"=0.0, "IBP1"=0.0, "IBP2"=0.0}} ("Data"), "Gradients"=w411, "ECG"=w409, "IBP"=w395) -> (w410:T16)
        n252 = case shown="True" w428 {
          tunnel: w429 -> [_ w523]
          tunnel: w410 -> [_ w521]
          frame False {
          }
          frame True {
            n253 = xnode ("FIFO Write")("Element"=w521, "Timeout"=0, "FIFO In"=w523) -> ()  [unwired: 2 out]
          }
        }
        n254 = Fixed-Point to Integer Cast(1:w396) -> (0:w405:i16)
        n255 = Fixed-Point to Integer Cast(1:w394) -> (0:w406:i16)
        n256 = local write "IPB0 In"(w405) -> ()
        n257 = local write "IBP1 In"(w406) -> ()
      }
    }
    n258 = Equal To 0?(x=w374) -> (x = 0?=w373:bool)
    n259 = local read "Stop"() -> (w372:bool)
  }
  n260 = node-c288 ("Output Node")(w27) -> ()
  n261 = node-c288(w2) -> ()
  n262 = disable-structure shown="Disabled" {
    frame Disabled {
      w524 = TRUE
      n263 = xnode ("PWMIO")("Connector2/DIO2"=w524, "Connector2/DIO3"=w524, "Connector2/DIO4"=w524, "Connector2/DIO5"=w524) -> ()  [unwired: 4 in, 4 out]
    }
    frame Enabled {
    }
  }
  n264 = Initialize Array(FALSE, 128 ("dimension size")) -> (w25:bool[])
  n265 = while {
    tunnel: w25 -> [w526]
    tunnel: w5 -> [_]
    stop <- w525 stop-if-true
    # "SPI Interface\nThis code reads in the SPI interface data and coverts it to integer data for processing"
    n266 = xnode "FPGA I/O Node"() -> ("FPGA I/O Out"=w527:refnum<k21>)  [unwired: 1 in, 1 out]
    n267 = xnode "FPGA I/O Method Node"("FPGA I/O In"=w527, "Timeout"=-1) -> ("Timed Out"=w528:bool)  [unwired: 1 out]
    n268 = case shown="False" w528 {
      tunnel: w526 -> [w561 _]
      frame False {
        w557 = FALSE
        n269 = node-c288() -> (w560:T6)  [unwired: 1 in]
        n270 = timed-loop {
          shift-right: [w573] -> w556
          shift-left: w561 -> [w574]
          timing: w560 -> [_]
          timing-out: [_] -> w559
          shift-right: [w569] -> _
          shift-left: w557 -> [w572]
          shift-right: [w570] -> _
          shift-left: u8 0 -> [w571]
          shift-left: w557 -> [w565]
          shift-left: w557 -> [w564]
          shift-left: w557 -> [w563]
          shift-left: w557 -> [w562]
          stop <- w575 stop-if-true
          n271 = xnode "FPGA I/O Node"() -> ("MOSI"=w566:bool)  [unwired: 1 in, 1 out]
          n272 = xnode "FPGA I/O Node"() -> ("SCLK"=w568:bool)  [unwired: 1 in, 1 out]
          n273 = Compound Arithmetic op=AND(invert w568, invert w572, invert w565, invert w564, invert w563, w562) -> (w567:bool)
          n274 = case shown="True" w567 {
            tunnel: [FALSE w586] -> w575
            tunnel: w574 -> [w576 w585]
            tunnel: [w576 w584] -> w573
            tunnel: w571 -> [w579 w583]
            tunnel: [w579 w582] -> w570
            tunnel: w568 -> [w578 w581]
            tunnel: [w578 w581] -> w569
            tunnel: w566 -> [_ w580]
            frame False {
            }
            frame True {
              n275 = Increment(x=w583) -> (x+1=w582:u8)
              n276 = xnode "FPGA I/O Node"("MOSI Data"=w580) -> ()  [unwired: 1 in, 1 out]
              n277 = Replace Array Subset(array=w585, new element=w580, index=w583) -> (w584:bool[])
              n278 = Equal?(x=u8 127, y=w583) -> (x = y?=w586:bool)
            }
          }
          n279 = xnode "FPGA I/O Node"("MOSI Out"=w566, "SCLK Edge"=w567, "SCLK Out"=w568) -> ()  [unwired: 3 in, 3 out]
        }
        n280 = node-c288(w559) -> ()
        n281 = call "Convert SPI Data to Numbers.vi"("Data In"=w556) -> ("IBP Data"=w536:T4, "ECG Data"=w547:T5)
        "ECG Data" <- w547
        "IBP Data" <- w536
        n282 = Unbundle By Name(w536) -> ("IBP0"=w535:fxp<+/-,16,16>, "IBP1"=w533:fxp<+/-,16,16>, "IBP2"=w531:fxp<+/-,16,16>)
        n283 = Unbundle By Name(w547) -> ("RA"=w555:fxp<+/-,16,16>, "LA"=w554:fxp<+/-,16,16>, "LL"=w553:fxp<+/-,16,16>, "V1"=w552:fxp<+/-,16,16>, "V2"=w551:fxp<+/-,16,16>, "V3"=w550:fxp<+/-,16,16>, "V4"=w549:fxp<+/-,16,16>, "V5"=w548:fxp<+/-,16,16>, "V6"=w538:fxp<+/-,16,16>)
        n284 = Fixed-Point to Integer Cast(1:w555) -> (0:→"RA":i16)
        n285 = Fixed-Point to Integer Cast(1:w554) -> (0:→"LA":i16)
        n286 = Fixed-Point to Integer Cast(1:w553) -> (0:→"LL":i16)
        n287 = Fixed-Point to Integer Cast(1:w552) -> (0:→"V1":i16)
        n288 = Fixed-Point to Integer Cast(1:w551) -> (0:→"V2":i16)
        n289 = Fixed-Point to Integer Cast(1:w550) -> (0:→"V3":i16)
        n290 = Fixed-Point to Integer Cast(1:w549) -> (0:→"V4":i16)
        n291 = Fixed-Point to Integer Cast(1:w548) -> (0:→"V5":i16)
        n292 = Fixed-Point to Integer Cast(1:w538) -> (0:→"V6":i16)
        n293 = Fixed-Point to Integer Cast(1:w535) -> (0:→"IBP0":i16)
        n294 = Fixed-Point to Integer Cast(1:w533) -> (0:→"IBP1":i16)
        n295 = Fixed-Point to Integer Cast(1:w531) -> (0:→"IBP2":i16)
      }
      frame True {
      }
    }
    n296 = local read "Stop"() -> (w525:bool)
  }
  n297 = while {
    tunnel: w10 -> [w605]
    tunnel: refnum<k21> "IO Taps 0" ("Memory") -> [w604]
    tunnel: refnum<k21> "IO Weights 0" ("Memory In") -> [w603]
    tunnel: refnum<k21> "IO Taps 1" ("Memory") -> [w602]
    tunnel: refnum<k21> "IO Weights 1" ("Memory In") -> [w601]
    tunnel: refnum<k21> "IO Taps 2" ("Memory") -> [w600]
    tunnel: refnum<k21> "IO Weights 2" ("Memory In") -> [w599]
    tunnel: refnum<k21> "IO Taps 3" ("Memory") -> [w598]
    tunnel: refnum<k21> "IO Weights 3" ("Memory In") -> [w597]
    tunnel: refnum<k21> "IO Taps 4" ("Memory") -> [w596]
    tunnel: refnum<k21> "IO Weights 4" ("Memory In") -> [w595]
    tunnel: refnum<k21> "IO Taps 5" ("Memory") -> [w594]
    tunnel: refnum<k21> "IO Weights 5" ("Memory In") -> [w593]
    tunnel: w5 -> [_]
    stop <- w592 stop-if-true
    # "Taps and Weights\nThis code reads memory blocks that keep the taps and weights data for the LMS adaptive filter of each ECG channel and exports the data via\nFIFO to the host machine"
    n298 = local read "Send"() -> (w606:bool)
    n299 = case shown="True" w606 {
      selector: w606 -> [_ w632]
      tunnel: w605 -> [_ w630]
      tunnel: w604 -> [_ w628]
      tunnel: w603 -> [_ w627]
      tunnel: w602 -> [_ w624]
      tunnel: w601 -> [_ w623]
      tunnel: w600 -> [_ w621]
      tunnel: w599 -> [_ w620]
      tunnel: w598 -> [_ w616]
      tunnel: w597 -> [_ w615]
      tunnel: w596 -> [_ w610]
      tunnel: w595 -> [_ w609]
      tunnel: w594 -> [_ w608]
      tunnel: w593 -> [_ w607]
      frame False {
      }
      frame True {
        n300 = Not(x=w632) -> (.not. x?=w631:bool)
        n301 = call "Stream Taps Data.vi"("FIFO In"=w630, "Memory"=w628) -> ("FIFO out"=w629:refnum<k21>)
        n302 = local write "Send"(w631) -> ()
        n303 = call "Stream Weights Output.vi"("FIFO in"=w629, "Memory In"=w627) -> ("FIFO out"=w625:refnum<k21>)
        n304 = call "Stream Taps Data.vi"("FIFO In"=w625, "Memory"=w624) -> ("FIFO out"=w626:refnum<k21>)
        n305 = call "Stream Weights Output.vi"("FIFO in"=w626, "Memory In"=w623) -> ("FIFO out"=w622:refnum<k21>)
        n306 = call "Stream Taps Data.vi"("FIFO In"=w622, "Memory"=w621) -> ("FIFO out"=w619:refnum<k21>)
        n307 = call "Stream Weights Output.vi"("FIFO in"=w619, "Memory In"=w620) -> ("FIFO out"=w618:refnum<k21>)
        n308 = call "Stream Taps Data.vi"("FIFO In"=w618, "Memory"=w616) -> ("FIFO out"=w617:refnum<k21>)
        n309 = call "Stream Weights Output.vi"("FIFO in"=w617, "Memory In"=w615) -> ("FIFO out"=w611:refnum<k21>)
        n310 = call "Stream Taps Data.vi"("FIFO In"=w611, "Memory"=w610) -> ("FIFO out"=w612:refnum<k21>)
        n311 = call "Stream Weights Output.vi"("FIFO in"=w612, "Memory In"=w609) -> ("FIFO out"=w613:refnum<k21>)
        n312 = call "Stream Taps Data.vi"("FIFO In"=w613, "Memory"=w608) -> ("FIFO out"=w614:refnum<k21>)
        n313 = call "Stream Weights Output.vi"("FIFO in"=w614, "Memory In"=w607) -> ()  [unwired: 1 out]
      }
    }
    n314 = local read "Stop"() -> (w592:bool)
  }
